vi "Jog.vi"(9 "Jog":T1={"X-"=FALSE, "X+"=FALSE, "Y-"=FALSE, "Y+"=FALSE, "Z_"=FALSE, "Z+"=FALSE, "Dist"=1000, "Feed"=500} {"Feed" items=["100 mm/min"=100, "200 mm/min"=200, "300 mm/min"=300, "400 mm/min"=400, "500 mm/min"=500]; "Dist" items=["0.1 mm"=1, "1 mm"=10, "10 mm"=100, "100 mm"=1000]}) -> (0 "Commands":string[](array[string]), 2 "resulting string":string, 3 "output cluster":T1)   [LabVIEW 2024]
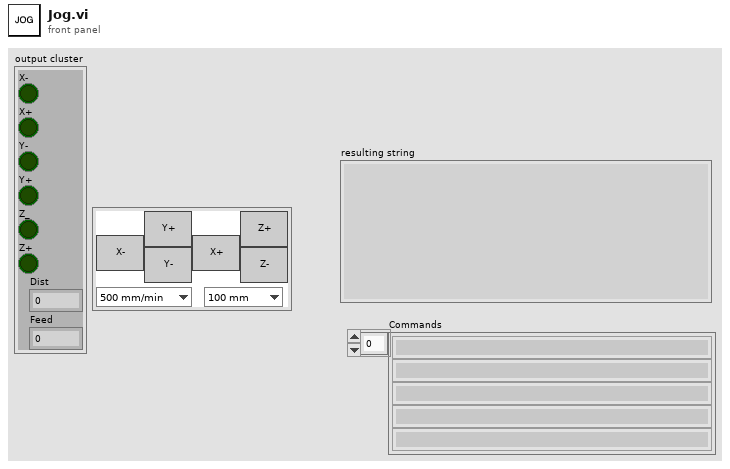
[diagram p1: front panel]
types:
  T1 = cluster{"X-":bool, "X+":bool, "Y-":bool, "Y+":bool, "Z_":bool, "Z+":bool, "Dist":u16, "Feed":u16}
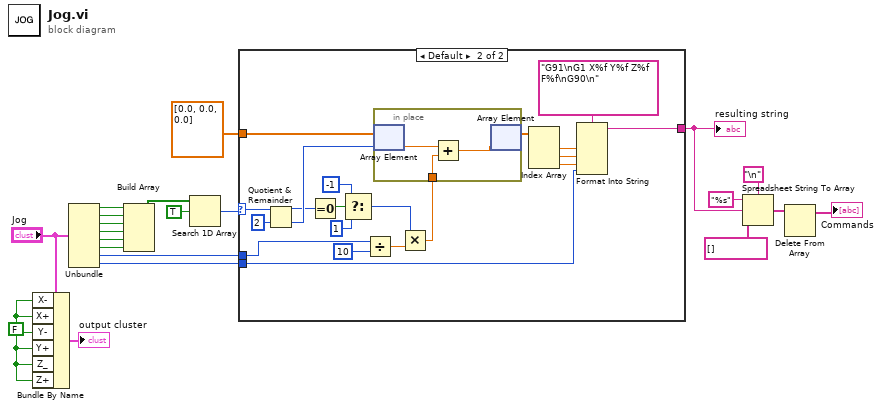
[diagram p0: block diagram]
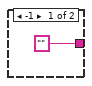
[diagram p2: hidden frame]
diagram:
  w3 = FALSE
  n1 = Bundle By Name(cluster="Jog", "X-"=w3, "X+"=w3, "Y-"=w3, "Y+"=w3, "Z_"=w3, "Z+"=w3) -> (→"output cluster":T1)
  n2 = Unbundle("Jog") -> ("X-"=w20:bool, "X+"=w19:bool, "Y-"=w18:bool, "Y+"=w17:bool, "Z_"=w16:bool, "Z+"=w15:bool, "Dist"=w21:u16, "Feed"=w11:u16)
  n3 = Build Array(w20, w19, w18, w17, w16, w15) -> (w14:bool[])
  n4 = Search 1D Array(1D array=w14, element=TRUE) -> (index of element=w12:i32)  [unwired: 1 in]
  n5 = case shown="Default" w12 {
    selector: w12 -> [_ w42]
    tunnel: w21 -> [_ w30]
    tunnel: dbl[] [0.0, 0.0, 0.0] -> [_ w40]
    tunnel: w11 -> [_ w32]
    tunnel: ["" w31] -> w6
    frame -1 {
    }
    frame Default {
      n6 = Quotient & Remainder(x=w42, y=2) -> (x-y*floor(x/y)=w27:i32, floor(x/y)=w39:i32)
      n7 = Equal To 0?(x=w27) -> (x = 0?=w26:bool)
      n8 = Select(t=-1 ("y"), s=w26, f=1 ("y")) -> (s? t:f=w25:i32)
      n9 = Divide(x=w30, y=u16 10) -> (x/y=w29:dbl)
      n10 = Multiply(x=w25, y=w29) -> (x*y=w38:dbl)
      n11 = in-place {
        in-place-border: w38 -> [w45]
        n12 = in-place-array #1(w40, w39) -> (w44:dbl)
        n13 = Add(x=w44, y=w45) -> (x+y=w43:dbl)
        n14 = in-place-array #1(w43) -> (w37:dbl[])  [unwired: 1 out]
      }
      n15 = Index Array(array=w37) -> (element #1=w36:dbl, element #2=w33:dbl, element #3=w34:dbl)  [unwired: 3 in]
      n16 = Format Into String(format string="G91\nG1 X%f Y%f Z%f F%f\nG90\n" ("Value (Signaling)"), w36, w33, w34, w32) -> (resulting string=w31:string)  [unwired: 2 in, 1 out]
    }
  }
  "resulting string" <- w6
  n17 = Spreadsheet String To Array(delimiter (Tab)="\n", format string="%s", spreadsheet string=w6, array type (2D Dbl)=string[] []) -> (array=w5:string[])
  n18 = Delete From Array(array=w5) -> (array with subset deleted=→"Commands":string[])  [unwired: 2 in, 1 out]
